vi "Stop Task.vi"(8 "error in (no error)":errorcluster, 11 "Hardware Refs In":T1={"IP Address"="Simulator", "Handle"=0, "Refresh Time (ms)"=0.0}) -> (0 "error out":errorcluster)   [LabVIEW 2013, in "Capacitive.lvlib"]
uses:
  Capacitive.lvlib
  Hardware Configuration.ctl
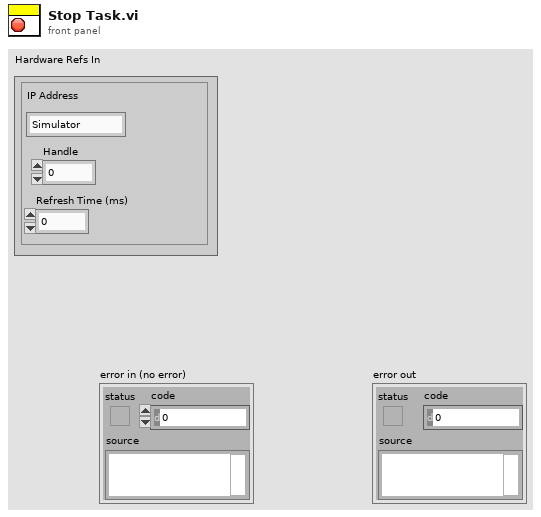
[diagram p1: front panel]
types:
  T1 = typedef "Capacitive.lvlib/Hardware Configuration.ctl" = cluster{"IP Address":string, "Handle":u32, "Refresh Time (ms)":dbl}
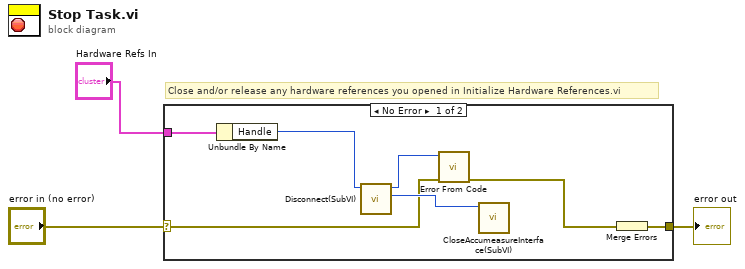
[diagram p0: block diagram]
diagram:
  # "Close and/or release any hardware references you opened in Initialize Hardware References.vi"
  n1 = case shown="No Error" "error in (no error)" {
    selector: "error in (no error)" -> [w5 w11]
    tunnel: [w10 w11] -> w2
    tunnel: "Hardware Refs In" -> [w9 _]
    frame No Error {
      n2 = Unbundle By Name(w9) -> ("Handle"=w8:u32)
      n3 = call "Disconnect(SubVI).vi"("Handle"=w8) -> ("Handle"=w7:u32, "Status"=w6:i32)  [unwired: 9 in]
      n4 = call "Error From Code.vi"("error in (no error)"=w5, "ErrorCode"=w6) -> ("error out"=w4:errorcluster)  [unwired: 9 in]
      n5 = call "CloseAccumeasureInterface(SubVI).vi"("Handle"=w7) -> ()  [unwired: 11 in]
      n6 = Merge Errors(w4) -> (w10:errorcluster)
    }
    frame Error {
    }
  }
  "error out" <- w2
